vi "6-c.vi"() -> ()   [LabVIEW 2017]
panel:
  in  "停止":bool
  out "波形图表":dbl(graph)
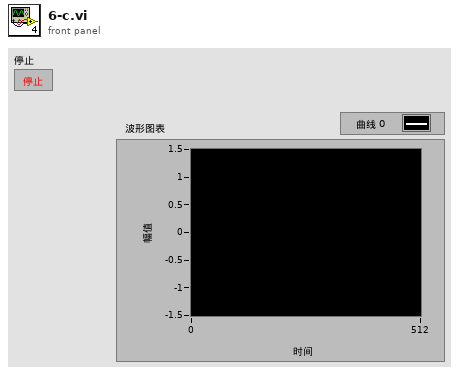
[diagram p1: front panel]
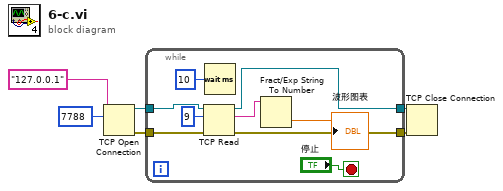
[diagram p0: block diagram]
diagram:
  n1 = TCP Open Connection(address="127.0.0.1" ("地址"), remote port or service name=u16 7788 ("远程端口或服务名称")) -> (connection ID=w6:refnum<k5>, error out=w5:errorcluster)  [unwired: 3 in]
  n2 = while {
    tunnel: w6 -> [w14]
    tunnel: w5 -> [w13]
    tunnel: [w12] -> w4
    tunnel: [w11] -> w3
    stop <- "停止" stop-if-true
    n3 = TCP Read(connection ID=w14, bytes to read=9 ("读取的字节"), error in (no error)=w13) -> (connection ID out=w12:refnum<k5>, data out=w10:string, error out=w11:errorcluster)  [unwired: 2 in]
    n4 = Wait (ms)(milliseconds to wait=u32 10 ("等待时间（毫秒）")) -> ()  [unwired: 1 out]
    n5 = Fract/Exp String To Number(string=w10) -> (number=→"波形图表":dbl)  [unwired: 3 in, 1 out]
  }
  n6 = TCP Close Connection(connection ID=w4, error in (no error)=w3) -> ()  [unwired: 1 in, 2 out]
